vi "Save Specific Configuration.vi"(8 "error in":errorcluster) -> (0 "error out":errorcluster, 3 "Cellular":string)   [LabVIEW 2021]
panel:
  in  "Cellular Technology":T1
  # "PLEASE SELECT THE TECHNOLOGY"
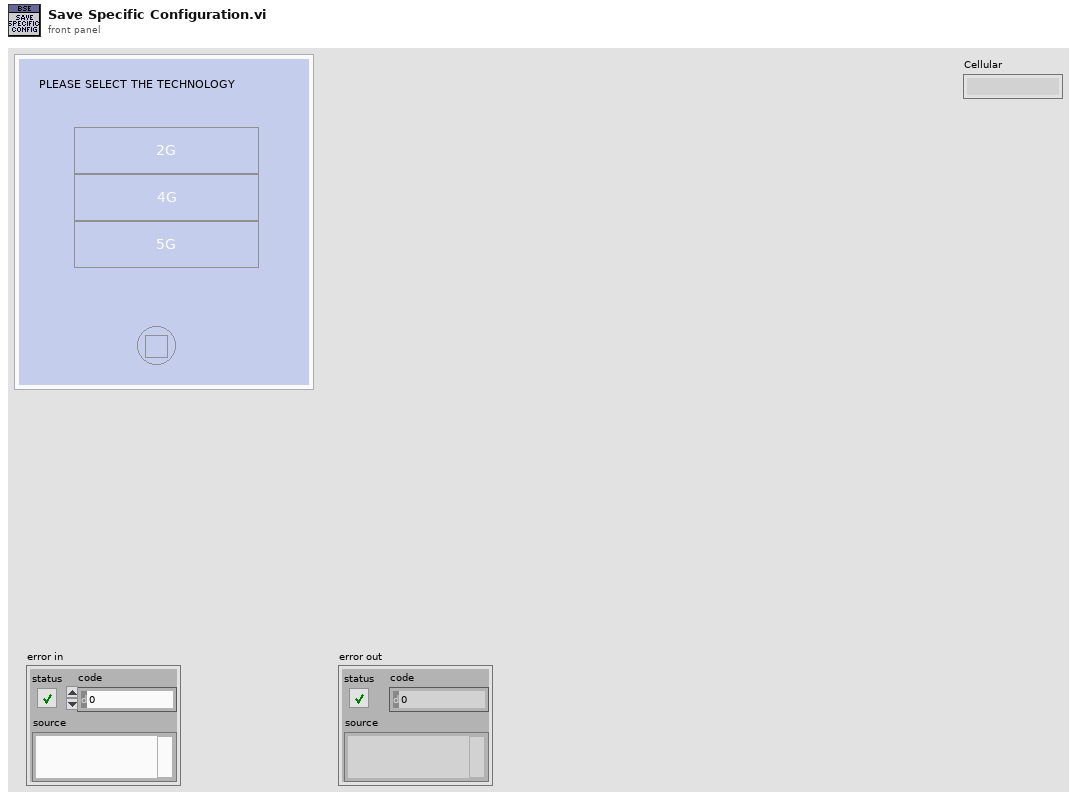
[diagram p1: front panel]
types:
  T1 = cluster{"OK":bool, "2G":bool, "5G":bool, "4G":bool, "Status":string}
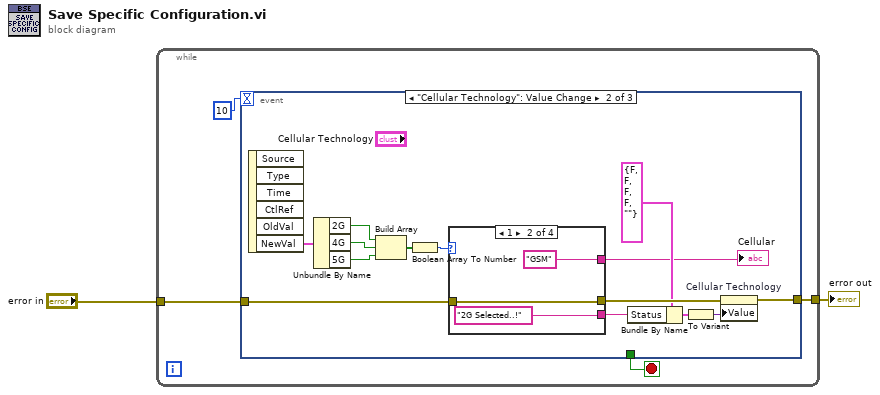
[diagram p0: block diagram]
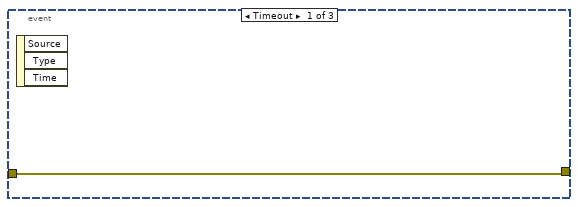
[diagram p2: hidden frame]
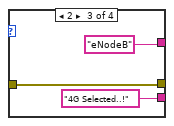
[diagram p4: hidden frame]
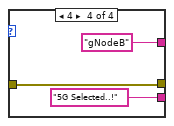
[diagram p5: hidden frame]
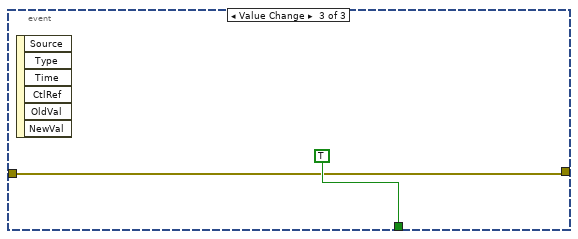
[diagram p6: hidden frame]
diagram:
  n1 = while {
    tunnel: "error in" -> [w4]
    tunnel: [w3] -> w2
    stop <- w5 stop-if-true
    n2 = event shown="[1] \"Cellular Technology\": Value Change" {
      selector: _ -> [_ _ _]
      dyn-events: _ -> [_ _ _]
      timeout: 10 -> [_ _ _]
      tunnel: [_ _ TRUE ("NewVal")] -> w5
      tunnel: w4 -> [w7 w15 w32]
      tunnel: [w7 w14 w32] -> w3
      event Timeout {
        n3 = event-data() -> ()  [unwired: 1 in, 3 out]
      }
      event "Cellular Technology": Value Change {
        n4 = event-data() -> ("NewVal"=w17:T1)  [unwired: 1 in, 5 out]
        n5 = Unbundle By Name(w17) -> ("2G"=w21:bool, "4G"=w20:bool, "5G"=w19:bool)
        n6 = Build Array(w21, w20, w19) -> (w18:bool[])
        n7 = Boolean Array To Number(Boolean array=w18) -> (number=w16:u32)
        n8 = case shown="1" w16 {
          tunnel: w15 -> [w22 w24 w27 w30]
          tunnel: [_ "2G Selected..!" "4G Selected..!" "5G Selected..!"] -> w11
          tunnel: [w22 w24 w27 w30] -> w12
          tunnel: [_ "GSM" "eNodeB" "gNodeB"] -> w8
          frame Default {
          }
          frame 1 {
          }
          frame 2 {
          }
          frame 4 {
          }
        }
        "Cellular" <- w8
        n9 = Bundle By Name(cluster=T1 {"OK"=FALSE, "2G"=FALSE, "5G"=FALSE, "4G"=FALSE, "Status"=""} ("Cellular Technology"), "Status"=w11) -> (w10:T1)
        n10 = To Variant(anything=w10) -> (Variant=w13:variant)
        n11 = property on="Cellular Technology" class="Clust"(error in=w12, "Value"=w13) -> (error out=w14:errorcluster)  [unwired: 1 in, 1 out]
      }
      event "Cellular Technology.OK": Value Change {
        n12 = event-data() -> ()  [unwired: 1 in, 6 out]
      }
    }
  }
  "error out" <- w2
